vi "Odd.vi"() -> ()   [LabVIEW 2024]
uses:
  <vilib>/numeric/Random Number (Range) U64.vi
  <vilib>/numeric/sub_Random U32.vi
panel:
  out "Array":u64[](array[numeric])
  out "Array 2":dbl[](array[numeric])
  in  "Numeric":i32
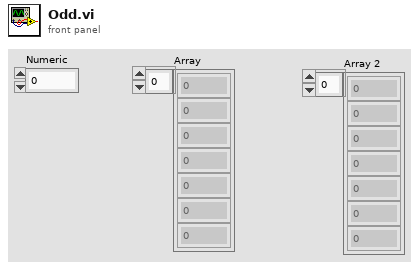
[diagram p1: front panel]
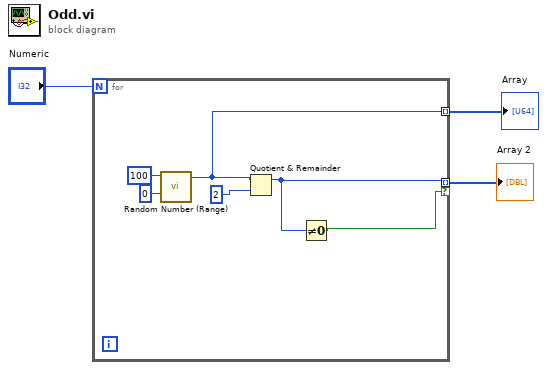
[diagram p0: block diagram]
diagram:
  n1 = for {
    N: "Numeric" -> [_]
    tunnel: [w4] -> w2 mode=indexing if=w7
    tunnel: [w5] -> w1 mode=indexing
    n2 = call-poly <vilib>:"Random Number (Range).vi"("lower bound (0)"=u64 0, "upper bound (100)"=u64 100) -> ("number"=w5:u64)  [unwired: 9 in]
    n3 = Quotient & Remainder(x=w5, y=u64 2) -> (x-y*floor(x/y)=w4:u64)  [unwired: 1 out]
    n4 = Not Equal To 0?(x=w4) -> (x != 0?=w7:bool)
  }
  "Array 2" <- w2
  "Array" <- w1
